vi "Power On (2-port).vi"(0 "Power Port in":refnum<visa-resource-name>="COM12", 7 "On/Off":enum16{"Power Off", "Power On"}(ring), 9 "Valid":bool[](array[boolean]), 11 "error in (no error)":errorcluster) -> (4 "Power Port out":refnum<visa-resource-name>="COM12", 15 "error out":errorcluster)   [LabVIEW 2010]
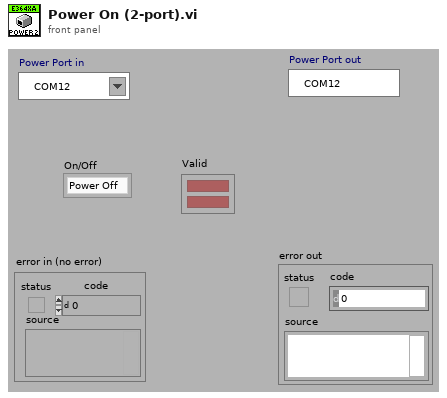
[diagram p1: front panel]
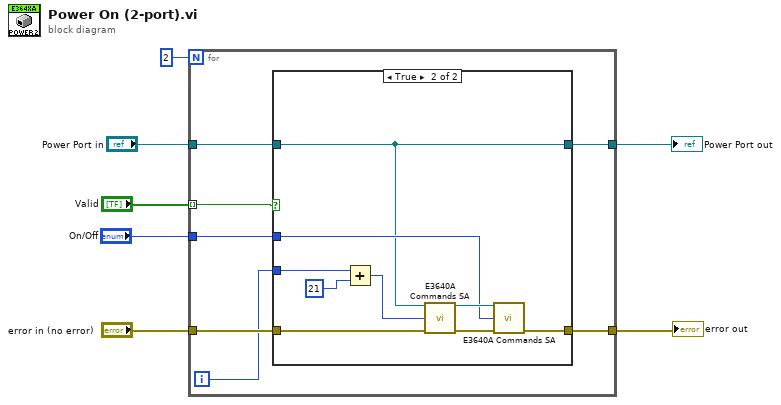
[diagram p0: block diagram]
diagram:
  n1 = for {
    N: 2 -> [_]
    tunnel: "error in (no error)" -> [w14]
    tunnel: "Power Port in" -> [w13]
    tunnel: "Valid" -> [w12] mode=indexing
    tunnel: [w11] -> w3
    tunnel: [w10] -> w2
    tunnel: "On/Off" -> [w9]
    i -> [w8]
    n2 = case shown="True" w12 {
      tunnel: w14 -> [w16 w25]
      tunnel: w13 -> [w15 w17]
      tunnel: [w15 w17] -> w11
      tunnel: [w16 w22] -> w10
      tunnel: w9 -> [_ w19]
      tunnel: w8 -> [_ w18]
      frame False {
      }
      frame True {
        n3 = Add(x=w18, y=21) -> (x+y=w24:i32)
        n4 = call "E3640A Commands SA.vi"("VISA session"=w17, "Command"=w24, "error in (no error)"=w25) -> ("VISA session out"=w20:refnum<visa-resource-name>, "error out"=w21:errorcluster)  [unwired: 7 in, 4 out]
        n5 = call "E3640A Commands SA.vi"("VISA session"=w20, "Command"=w19, "error in (no error)"=w21) -> ("error out"=w22:errorcluster)  [unwired: 7 in, 5 out]
      }
    }
  }
  "error out" <- w2
  "Power Port out" <- w3
